vi "DataSave.vi"(3 "Data":u32[](array[numeric]), 5 "File Refnum":refnum<file>) -> ()   [LabVIEW 2011]
panel:
  out "Data size":i32
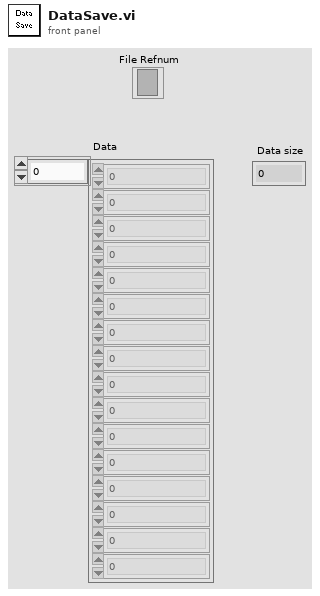
[diagram p1: front panel]
types:
  T1 = enum16{"big-endian, network order", "native, host order", "little-endian"}
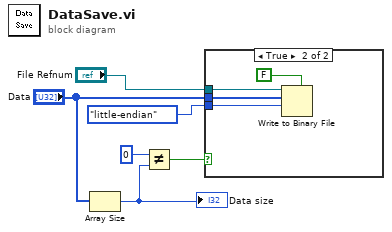
[diagram p0: block diagram]
diagram:
  n1 = Array Size(array="Data") -> (size(s)=w4:i32)
  "Data size" <- w4
  n2 = Not Equal?(x=0, y=w4) -> (x != y?=w3:bool)
  n3 = case shown="True" w3 {
    tunnel: "File Refnum" -> [_ w10]
    tunnel: "Data" -> [_ w9]
    tunnel: T1."little-endian" ("byte order (0:big-endian, network order)") -> [_ w8]
    frame False {
    }
    frame True {
      n4 = Write to Binary File(file (use dialog)=w10, data=w9, 5:FALSE ("prepend array or string size? (T)"), 9:w8) -> ()  [unwired: 2 in, 3 out]
    }
  }
